vi "Target4.vi"   [LabVIEW 2025]
uses:
  <vilib>/eio/utilities/niEioResolveVilibRelativePath.vi
  <vilib>/rvi/interface/RandomDataEmulation/niFpgaRandomDataHandleErrors.vi
  <vilib>/rvi/Memory/Memory_Emulation/nirvimemoryFastEmulation.vi
  <vilib>/rvi/Memory/Memory_Emulation/nirvimemoryEmulation.vi
  <vilib>/rvi/Emulation/niFpgaEmulationIsFPGAContextNoSignature.vi
  <vilib>/rvi/DataTransferAndStorage/Container/Common/niFpgaContainerGetUniqueNameForEmu.vi
  <vilib>/rvi/Emulation/niFpgaProcessEmulError.vi
  <vilib>/rvi/Emulation/niFpgaSctlEmulationGetInTimedLoop.vi
  <vilib>/rvi/errors/nirviReportUnexpectedCaseInternalError (U32).vi
  <vilib>/rvi/DataTransferAndStorage/Container/XNode/niFpgaContainer.xnode
  <vilib>/rvi/interface/RandomDataEmulation/nirviRandomDataFpgaReadWriteTemplate.vi
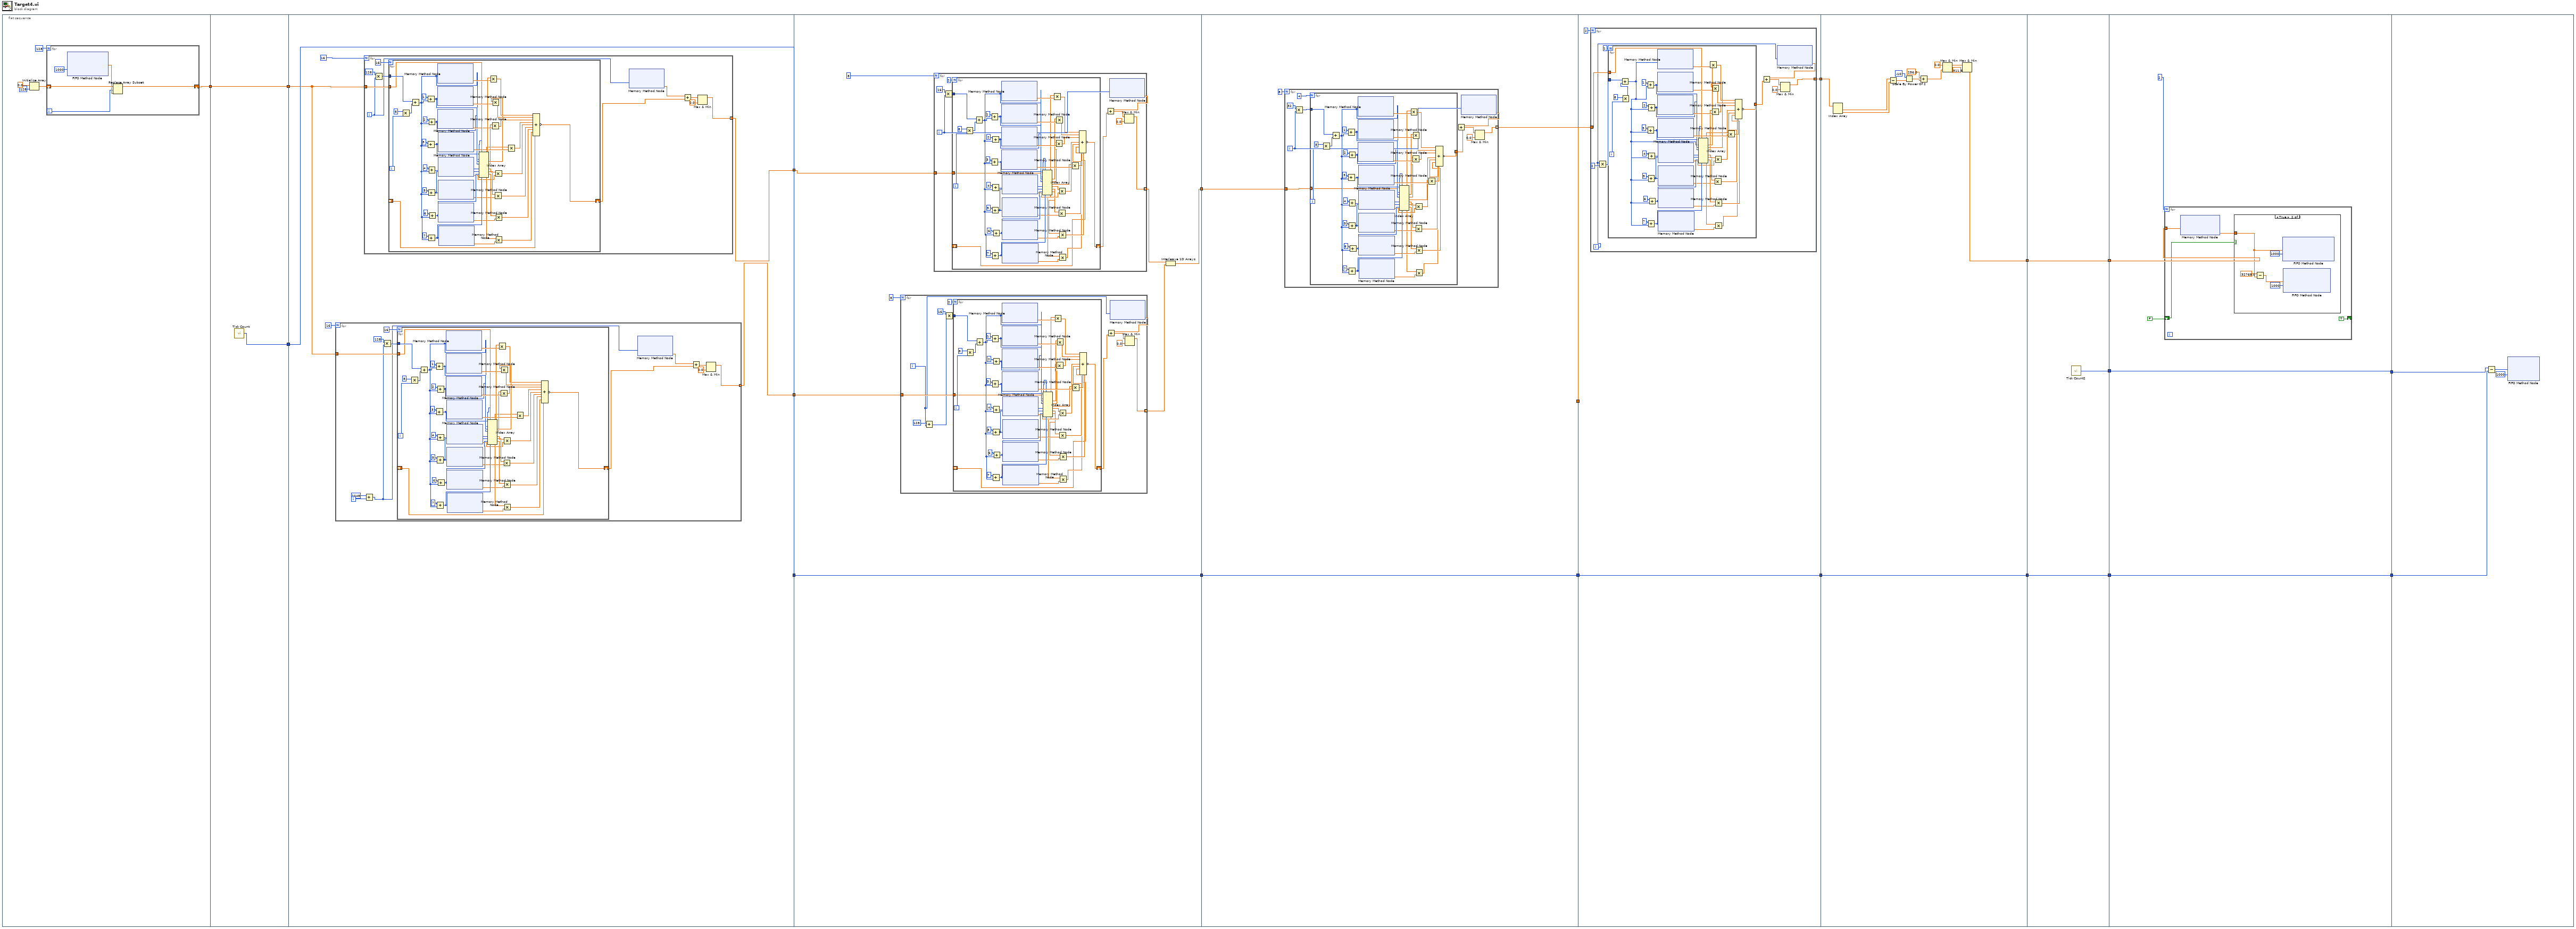
[diagram p0: block diagram]
diagram:
  n1 = flat-sequence {
    tunnel: [w23] -> w19
    tunnel: w19 -> [w31]
    tunnel: [w31] -> w18
    tunnel: [w30] -> w17
    tunnel: w18 -> [w34]
    tunnel: w17 -> [w36]
    tunnel: [w36] -> w7
    tunnel: [w33] -> w2
    tunnel: [w32] -> w1
    tunnel: w7 -> [w159]
    tunnel: [w159] -> w5
    tunnel: [w156] -> w3
    tunnel: w2 -> [w153]
    tunnel: w1 -> [w152]
    tunnel: [w275] -> w6
    tunnel: w5 -> [w277]
    tunnel: [w277] -> w4
    tunnel: w3 -> [w274]
    tunnel: w6 -> [w335]
    tunnel: [w334] -> w16
    tunnel: [w336] -> w8
    tunnel: w4 -> [w336]
    tunnel: w16 -> [w394]
    tunnel: [w396] -> w15
    tunnel: [w395] -> w9
    tunnel: w8 -> [w395]
    tunnel: w15 -> [w407]
    tunnel: [w407] -> w14
    tunnel: [w406] -> w13
    tunnel: [w405] -> w10
    tunnel: w9 -> [w405]
    tunnel: w14 -> [w411]
    tunnel: [w409] -> w12
    tunnel: w13 -> [w409]
    tunnel: [w408] -> w11
    tunnel: w10 -> [w408]
    tunnel: w12 -> [w425]
    tunnel: w11 -> [w422]
    frame #0 {
      n2 = Initialize Array(sgl 0.0 ("element"), 128 ("dimension size")) -> (w20:sgl[])
      n3 = for {
        N: 128 -> [_]
        shift-right: [w26] -> w23
        shift-left: w20 -> [w28]
        i -> [w25]
        n4 = xnode ("FIFO Method Node")("Timeout"=1000) -> ("Element"=w27:sgl)  [unwired: 1 in, 2 out]
        n5 = Replace Array Subset(array=w28, new element=w27, index=w25) -> (w26:sgl[])
      }
    }
    frame #1 {
      n6 = call "Tick Count"() -> ("Tick Count(uSec)"=w30:u32)
    }
    frame #2 {
      n7 = for {
        N: 16 -> [_]
        tunnel: w34 -> [w44]
        tunnel: [w43] -> w32 mode=indexing
        i -> [w40]
        n8 = Add(x=2048, y=w40) -> (x+y=w39:i32)
        n9 = Multiply(x=128, y=w39) -> (x*y=w47:i32)
        n10 = for {
          N: 16 -> [_]
          tunnel: w47 -> [w95]
          tunnel: w44 -> [w81]
          shift-right: [w50] -> w42
          shift-left: _ -> [w51]
          i -> [w94]
          n11 = Multiply(x=8, y=w94) -> (x*y=w92:i32)
          n12 = Add(x=w95, y=w92) -> (x+y=w56:i32)
          n13 = Add(x=1, y=w56) -> (x+y=w78:i32)
          n14 = Add(x=3, y=w56) -> (x+y=w74:i32)
          n15 = Add(x=5, y=w56) -> (x+y=w67:i32)
          n16 = Add(x=7, y=w56) -> (x+y=w65:i32)
          n17 = Add(x=2, y=w56) -> (x+y=w73:i32)
          n18 = Add(x=4, y=w56) -> (x+y=w68:i32)
          n19 = Add(x=6, y=w56) -> (x+y=w66:i32)
          n20 = xnode ("Memory Method Node")("Address"=w56) -> ("Data"=w87:sgl)  [unwired: 1 in, 1 out]
          n21 = xnode ("Memory Method Node")("Address"=w78) -> ("Data"=w82:sgl)  [unwired: 1 in, 1 out]
          n22 = xnode ("Memory Method Node")("Address"=w73) -> ("Data"=w79:sgl)  [unwired: 1 in, 1 out]
          n23 = xnode ("Memory Method Node")("Address"=w74) -> ("Data"=w80:sgl)  [unwired: 1 in, 1 out]
          n24 = xnode ("Memory Method Node")("Address"=w68) -> ("Data"=w57:sgl)  [unwired: 1 in, 1 out]
          n25 = xnode ("Memory Method Node")("Address"=w67) -> ("Data"=w58:sgl)  [unwired: 1 in, 1 out]
          n26 = xnode ("Memory Method Node")("Address"=w66) -> ("Data"=w59:sgl)  [unwired: 1 in, 1 out]
          n27 = xnode ("Memory Method Node")("Address"=w65) -> ("Data"=w60:sgl)  [unwired: 1 in, 1 out]
          n28 = Index Array(array=w81, index #1=w56, index #2=w78, index #3=w73, index #4=w74, index #5=w68, index #6=w67, index #7=w66, index #8=w65) -> (element #1=w88:sgl, element #2=w77:sgl, element #3=w76:sgl, element #4=w75:sgl, element #5=w64:sgl, element #6=w63:sgl, element #7=w62:sgl, element #8=w61:sgl)
          n29 = Multiply(x=w88, y=w87) -> (x*y=w86:sgl)
          n30 = Multiply(x=w76, y=w79) -> (x*y=w84:sgl)
          n31 = Multiply(x=w77, y=w82) -> (x*y=w85:sgl)
          n32 = Multiply(x=w63, y=w58) -> (x*y=w54:sgl)
          n33 = Multiply(x=w64, y=w57) -> (x*y=w55:sgl)
          n34 = Multiply(x=w62, y=w59) -> (x*y=w53:sgl)
          n35 = Multiply(x=w61, y=w60) -> (x*y=w52:sgl)
          n36 = Multiply(x=w75, y=w80) -> (x*y=w83:sgl)
          n37 = Compound Arithmetic op=ADD(w86, w85, w84, w83, w55, w54, w53, w52, w51) -> (invert w50:sgl)
        }
        n38 = xnode ("Memory Method Node")("Address"=w39) -> ("Data"=w41:sgl)  [unwired: 1 in, 1 out]
        n39 = Add(x=w41, y=w42) -> (x+y=w46:sgl)
        n40 = Max & Min(x=w46, y=sgl 0.0) -> (max(x,y)=w43:sgl)  [unwired: 1 out]
      }
      n41 = for {
        N: 16 -> [_]
        tunnel: w34 -> [w100]
        tunnel: [w98] -> w33 mode=indexing
        i -> [w99]
        n42 = Multiply(x=128, y=w99) -> (x*y=w103:i32)
        n43 = for {
          N: 16 -> [_]
          tunnel: w103 -> [w151]
          tunnel: w100 -> [w137]
          shift-right: [w106] -> w97
          shift-left: _ -> [w107]
          i -> [w150]
          n44 = Multiply(x=8, y=w150) -> (x*y=w148:i32)
          n45 = Add(x=w151, y=w148) -> (x+y=w112:i32)
          n46 = Add(x=1, y=w112) -> (x+y=w134:i32)
          n47 = Add(x=3, y=w112) -> (x+y=w130:i32)
          n48 = Add(x=5, y=w112) -> (x+y=w123:i32)
          n49 = Add(x=7, y=w112) -> (x+y=w121:i32)
          n50 = Add(x=2, y=w112) -> (x+y=w129:i32)
          n51 = Add(x=4, y=w112) -> (x+y=w124:i32)
          n52 = Add(x=6, y=w112) -> (x+y=w122:i32)
          n53 = xnode ("Memory Method Node")("Address"=w112) -> ("Data"=w143:sgl)  [unwired: 1 in, 1 out]
          n54 = xnode ("Memory Method Node")("Address"=w134) -> ("Data"=w138:sgl)  [unwired: 1 in, 1 out]
          n55 = xnode ("Memory Method Node")("Address"=w129) -> ("Data"=w135:sgl)  [unwired: 1 in, 1 out]
          n56 = xnode ("Memory Method Node")("Address"=w130) -> ("Data"=w136:sgl)  [unwired: 1 in, 1 out]
          n57 = xnode ("Memory Method Node")("Address"=w124) -> ("Data"=w113:sgl)  [unwired: 1 in, 1 out]
          n58 = xnode ("Memory Method Node")("Address"=w123) -> ("Data"=w114:sgl)  [unwired: 1 in, 1 out]
          n59 = xnode ("Memory Method Node")("Address"=w122) -> ("Data"=w115:sgl)  [unwired: 1 in, 1 out]
          n60 = xnode ("Memory Method Node")("Address"=w121) -> ("Data"=w116:sgl)  [unwired: 1 in, 1 out]
          n61 = Index Array(array=w137, index #1=w112, index #2=w134, index #3=w129, index #4=w130, index #5=w124, index #6=w123, index #7=w122, index #8=w121) -> (element #1=w144:sgl, element #2=w133:sgl, element #3=w132:sgl, element #4=w131:sgl, element #5=w120:sgl, element #6=w119:sgl, element #7=w118:sgl, element #8=w117:sgl)
          n62 = Multiply(x=w144, y=w143) -> (x*y=w142:sgl)
          n63 = Multiply(x=w132, y=w135) -> (x*y=w140:sgl)
          n64 = Multiply(x=w133, y=w138) -> (x*y=w141:sgl)
          n65 = Multiply(x=w119, y=w114) -> (x*y=w110:sgl)
          n66 = Multiply(x=w120, y=w113) -> (x*y=w111:sgl)
          n67 = Multiply(x=w118, y=w115) -> (x*y=w109:sgl)
          n68 = Multiply(x=w117, y=w116) -> (x*y=w108:sgl)
          n69 = Multiply(x=w131, y=w136) -> (x*y=w139:sgl)
          n70 = Compound Arithmetic op=ADD(w142, w141, w140, w139, w111, w110, w109, w108, w107) -> (invert w106:sgl)
        }
        n71 = xnode ("Memory Method Node")("Address"=w99) -> ("Data"=w96:sgl)  [unwired: 1 in, 1 out]
        n72 = Add(x=w96, y=w97) -> (x+y=w102:sgl)
        n73 = Max & Min(x=w102, y=sgl 0.0) -> (max(x,y)=w98:sgl)  [unwired: 1 out]
      }
    }
    frame #3 {
      n74 = for {
        N: 8 -> [_]
        tunnel: w152 -> [w165]
        tunnel: [w164] -> w154 mode=indexing
        i -> [w160]
        n75 = Add(x=128, y=w160) -> (x+y=w161:i32)
        n76 = Multiply(x=16, y=w161) -> (x*y=w168:i32)
        n77 = for {
          N: 2 -> [_]
          tunnel: w168 -> [w217]
          tunnel: w165 -> [w182]
          shift-right: [w173] -> w163
          shift-left: _ -> [w172]
          i -> [w216]
          n78 = Multiply(x=8, y=w216) -> (x*y=w214:i32)
          n79 = Add(x=w217, y=w214) -> (x+y=w183:i32)
          n80 = Add(x=1, y=w183) -> (x+y=w202:i32)
          n81 = Add(x=3, y=w183) -> (x+y=w201:i32)
          n82 = Add(x=5, y=w183) -> (x+y=w194:i32)
          n83 = Add(x=7, y=w183) -> (x+y=w192:i32)
          n84 = Add(x=2, y=w183) -> (x+y=w200:i32)
          n85 = Add(x=4, y=w183) -> (x+y=w195:i32)
          n86 = Add(x=6, y=w183) -> (x+y=w193:i32)
          n87 = xnode ("Memory Method Node")("Address"=w183) -> ("Data"=w210:sgl)  [unwired: 1 in, 1 out]
          n88 = xnode ("Memory Method Node")("Address"=w202) -> ("Data"=w205:sgl)  [unwired: 1 in, 1 out]
          n89 = xnode ("Memory Method Node")("Address"=w200) -> ("Data"=w203:sgl)  [unwired: 1 in, 1 out]
          n90 = xnode ("Memory Method Node")("Address"=w201) -> ("Data"=w204:sgl)  [unwired: 1 in, 1 out]
          n91 = xnode ("Memory Method Node")("Address"=w195) -> ("Data"=w188:sgl)  [unwired: 1 in, 1 out]
          n92 = xnode ("Memory Method Node")("Address"=w194) -> ("Data"=w189:sgl)  [unwired: 1 in, 1 out]
          n93 = xnode ("Memory Method Node")("Address"=w193) -> ("Data"=w190:sgl)  [unwired: 1 in, 1 out]
          n94 = xnode ("Memory Method Node")("Address"=w192) -> ("Data"=w191:sgl)  [unwired: 1 in, 1 out]
          n95 = Index Array(array=w182, index #1=w183, index #2=w202, index #3=w200, index #4=w201, index #5=w195, index #6=w194, index #7=w193, index #8=w192) -> (element #1=w181:sgl, element #2=w180:sgl, element #3=w179:sgl, element #4=w177:sgl, element #5=w178:sgl, element #6=w176:sgl, element #7=w175:sgl, element #8=w174:sgl)
          n96 = Multiply(x=w181, y=w210) -> (x*y=w209:sgl)
          n97 = Multiply(x=w179, y=w203) -> (x*y=w207:sgl)
          n98 = Multiply(x=w180, y=w205) -> (x*y=w208:sgl)
          n99 = Multiply(x=w176, y=w189) -> (x*y=w186:sgl)
          n100 = Multiply(x=w178, y=w188) -> (x*y=w187:sgl)
          n101 = Multiply(x=w175, y=w190) -> (x*y=w185:sgl)
          n102 = Multiply(x=w174, y=w191) -> (x*y=w184:sgl)
          n103 = Multiply(x=w177, y=w204) -> (x*y=w206:sgl)
          n104 = Compound Arithmetic op=ADD(w209, w208, w207, w206, w187, w186, w185, w184, w172) -> (invert w173:sgl)
        }
        n105 = xnode ("Memory Method Node")("Address"=w160) -> ("Data"=w170:sgl)  [unwired: 1 in, 1 out]
        n106 = Add(x=w170, y=w163) -> (x+y=w167:sgl)
        n107 = Max & Min(x=w167, y=sgl 0.0) -> (max(x,y)=w164:sgl)  [unwired: 1 out]
      }
      n108 = for {
        N: 8 -> [_]
        tunnel: w153 -> [w220]
        tunnel: [w219] -> w155 mode=indexing
        i -> [w224]
        n109 = Multiply(x=16, y=w224) -> (x*y=w223:i32)
        n110 = for {
          N: 2 -> [_]
          tunnel: w223 -> [w273]
          tunnel: w220 -> [w238]
          shift-right: [w229] -> w218
          shift-left: _ -> [w228]
          i -> [w272]
          n111 = Multiply(x=8, y=w272) -> (x*y=w270:i32)
          n112 = Add(x=w273, y=w270) -> (x+y=w239:i32)
          n113 = Add(x=1, y=w239) -> (x+y=w258:i32)
          n114 = Add(x=3, y=w239) -> (x+y=w257:i32)
          n115 = Add(x=5, y=w239) -> (x+y=w250:i32)
          n116 = Add(x=7, y=w239) -> (x+y=w248:i32)
          n117 = Add(x=2, y=w239) -> (x+y=w256:i32)
          n118 = Add(x=4, y=w239) -> (x+y=w251:i32)
          n119 = Add(x=6, y=w239) -> (x+y=w249:i32)
          n120 = xnode ("Memory Method Node")("Address"=w239) -> ("Data"=w266:sgl)  [unwired: 1 in, 1 out]
          n121 = xnode ("Memory Method Node")("Address"=w258) -> ("Data"=w261:sgl)  [unwired: 1 in, 1 out]
          n122 = xnode ("Memory Method Node")("Address"=w256) -> ("Data"=w259:sgl)  [unwired: 1 in, 1 out]
          n123 = xnode ("Memory Method Node")("Address"=w257) -> ("Data"=w260:sgl)  [unwired: 1 in, 1 out]
          n124 = xnode ("Memory Method Node")("Address"=w251) -> ("Data"=w244:sgl)  [unwired: 1 in, 1 out]
          n125 = xnode ("Memory Method Node")("Address"=w250) -> ("Data"=w245:sgl)  [unwired: 1 in, 1 out]
          n126 = xnode ("Memory Method Node")("Address"=w249) -> ("Data"=w246:sgl)  [unwired: 1 in, 1 out]
          n127 = xnode ("Memory Method Node")("Address"=w248) -> ("Data"=w247:sgl)  [unwired: 1 in, 1 out]
          n128 = Index Array(array=w238, index #1=w239, index #2=w258, index #3=w256, index #4=w257, index #5=w251, index #6=w250, index #7=w249, index #8=w248) -> (element #1=w237:sgl, element #2=w236:sgl, element #3=w235:sgl, element #4=w233:sgl, element #5=w234:sgl, element #6=w232:sgl, element #7=w231:sgl, element #8=w230:sgl)
          n129 = Multiply(x=w237, y=w266) -> (x*y=w265:sgl)
          n130 = Multiply(x=w235, y=w259) -> (x*y=w263:sgl)
          n131 = Multiply(x=w236, y=w261) -> (x*y=w264:sgl)
          n132 = Multiply(x=w232, y=w245) -> (x*y=w242:sgl)
          n133 = Multiply(x=w234, y=w244) -> (x*y=w243:sgl)
          n134 = Multiply(x=w231, y=w246) -> (x*y=w241:sgl)
          n135 = Multiply(x=w230, y=w247) -> (x*y=w240:sgl)
          n136 = Multiply(x=w233, y=w260) -> (x*y=w262:sgl)
          n137 = Compound Arithmetic op=ADD(w265, w264, w263, w262, w243, w242, w241, w240, w228) -> (invert w229:sgl)
        }
        n138 = xnode ("Memory Method Node")("Address"=w224) -> ("Data"=w226:sgl)  [unwired: 1 in, 1 out]
        n139 = Add(x=w226, y=w218) -> (x+y=w222:sgl)
        n140 = Max & Min(x=w222, y=sgl 0.0) -> (max(x,y)=w219:sgl)  [unwired: 1 out]
      }
      n141 = Interleave 1D Arrays(w155, w154) -> (w156:sgl[])
    }
    frame #4 {
      n142 = for {
        N: 8 -> [_]
        tunnel: [w280] -> w275 mode=indexing
        tunnel: w274 -> [w278]
        i -> [w284]
        n143 = Multiply(x=32, y=w284) -> (x*y=w283:i32)
        n144 = for {
          N: 4 -> [_]
          tunnel: w283 -> [w332]
          tunnel: [w317] -> w279
          tunnel: w278 -> [w296]
          i -> [w331]
          n145 = Multiply(x=8, y=w331) -> (x*y=w329:i32)
          n146 = Add(x=w332, y=w329) -> (x+y=w297:i32)
          n147 = Add(x=1, y=w297) -> (x+y=w316:i32)
          n148 = Add(x=3, y=w297) -> (x+y=w315:i32)
          n149 = Add(x=5, y=w297) -> (x+y=w308:i32)
          n150 = Add(x=7, y=w297) -> (x+y=w306:i32)
          n151 = Add(x=2, y=w297) -> (x+y=w314:i32)
          n152 = Add(x=4, y=w297) -> (x+y=w309:i32)
          n153 = Add(x=6, y=w297) -> (x+y=w307:i32)
          n154 = xnode ("Memory Method Node")("Address"=w297) -> ("Data"=w325:sgl)  [unwired: 1 in, 1 out]
          n155 = xnode ("Memory Method Node")("Address"=w316) -> ("Data"=w320:sgl)  [unwired: 1 in, 1 out]
          n156 = xnode ("Memory Method Node")("Address"=w314) -> ("Data"=w318:sgl)  [unwired: 1 in, 1 out]
          n157 = xnode ("Memory Method Node")("Address"=w315) -> ("Data"=w319:sgl)  [unwired: 1 in, 1 out]
          n158 = xnode ("Memory Method Node")("Address"=w309) -> ("Data"=w302:sgl)  [unwired: 1 in, 1 out]
          n159 = xnode ("Memory Method Node")("Address"=w308) -> ("Data"=w303:sgl)  [unwired: 1 in, 1 out]
          n160 = xnode ("Memory Method Node")("Address"=w307) -> ("Data"=w304:sgl)  [unwired: 1 in, 1 out]
          n161 = xnode ("Memory Method Node")("Address"=w306) -> ("Data"=w305:sgl)  [unwired: 1 in, 1 out]
          n162 = Index Array(array=w296, index #1=w297, index #2=w316, index #3=w314, index #4=w315, index #5=w309, index #6=w308, index #7=w307, index #8=w306) -> (element #1=w295:sgl, element #2=w294:sgl, element #3=w293:sgl, element #4=w292:sgl, element #5=w291:sgl, element #6=w290:sgl, element #7=w289:sgl, element #8=w288:sgl)
          n163 = Multiply(x=w295, y=w325) -> (x*y=w324:sgl)
          n164 = Multiply(x=w293, y=w318) -> (x*y=w322:sgl)
          n165 = Multiply(x=w294, y=w320) -> (x*y=w323:sgl)
          n166 = Multiply(x=w290, y=w303) -> (x*y=w300:sgl)
          n167 = Multiply(x=w291, y=w302) -> (x*y=w301:sgl)
          n168 = Multiply(x=w289, y=w304) -> (x*y=w299:sgl)
          n169 = Multiply(x=w288, y=w305) -> (x*y=w298:sgl)
          n170 = Multiply(x=w292, y=w319) -> (x*y=w321:sgl)
          n171 = Compound Arithmetic op=ADD(w324, w323, w322, w321, w301, w300, w299, w298) -> (invert w317:sgl)
        }
        n172 = xnode ("Memory Method Node")("Address"=w284) -> ("Data"=w286:sgl)  [unwired: 1 in, 1 out]
        n173 = Add(x=w286, y=w279) -> (x+y=w282:sgl)
        n174 = Max & Min(x=w282, y=sgl 0.0) -> (max(x,y)=w280:sgl)  [unwired: 1 out]
      }
    }
    frame #5 {
      n175 = for {
        N: 2 -> [_]
        tunnel: w335 -> [w346]
        tunnel: [w345] -> w334 mode=indexing
        i -> [w337]
        n176 = Multiply(x=w337, y=2) -> (x*y=w338:i32)
        n177 = for {
          N: 1 -> [_]
          tunnel: w346 -> [w379]
          tunnel: [w376] -> w340
          tunnel: w338 -> [w347]
          i -> [w391]
          n178 = Multiply(x=8, y=w391) -> (x*y=w349:i32)
          n179 = Add(x=w347, y=w349) -> (x+y=w348:i32)
          n180 = Add(x=1, y=w348) -> (x+y=w375:i32)
          n181 = Add(x=3, y=w348) -> (x+y=w371:i32)
          n182 = Add(x=5, y=w348) -> (x+y=w364:i32)
          n183 = Add(x=7, y=w348) -> (x+y=w362:i32)
          n184 = Add(x=2, y=w348) -> (x+y=w370:i32)
          n185 = Add(x=4, y=w348) -> (x+y=w365:i32)
          n186 = Add(x=6, y=w348) -> (x+y=w363:i32)
          n187 = xnode ("Memory Method Node")("Address"=w348) -> ("Data"=w385:sgl)  [unwired: 1 in, 1 out]
          n188 = xnode ("Memory Method Node")("Address"=w375) -> ("Data"=w380:sgl)  [unwired: 1 in, 1 out]
          n189 = xnode ("Memory Method Node")("Address"=w370) -> ("Data"=w377:sgl)  [unwired: 1 in, 1 out]
          n190 = xnode ("Memory Method Node")("Address"=w371) -> ("Data"=w378:sgl)  [unwired: 1 in, 1 out]
          n191 = xnode ("Memory Method Node")("Address"=w365) -> ("Data"=w354:sgl)  [unwired: 1 in, 1 out]
          n192 = xnode ("Memory Method Node")("Address"=w364) -> ("Data"=w355:sgl)  [unwired: 1 in, 1 out]
          n193 = xnode ("Memory Method Node")("Address"=w363) -> ("Data"=w356:sgl)  [unwired: 1 in, 1 out]
          n194 = xnode ("Memory Method Node")("Address"=w362) -> ("Data"=w357:sgl)  [unwired: 1 in, 1 out]
          n195 = Index Array(array=w379, index #1=w348, index #2=w375, index #3=w370, index #4=w371, index #5=w365, index #6=w364, index #7=w363, index #8=w362) -> (element #1=w386:sgl, element #2=w374:sgl, element #3=w373:sgl, element #4=w372:sgl, element #5=w361:sgl, element #6=w360:sgl, element #7=w359:sgl, element #8=w358:sgl)
          n196 = Multiply(x=w386, y=w385) -> (x*y=w384:sgl)
          n197 = Multiply(x=w373, y=w377) -> (x*y=w382:sgl)
          n198 = Multiply(x=w374, y=w380) -> (x*y=w383:sgl)
          n199 = Multiply(x=w360, y=w355) -> (x*y=w352:sgl)
          n200 = Multiply(x=w361, y=w354) -> (x*y=w353:sgl)
          n201 = Multiply(x=w359, y=w356) -> (x*y=w351:sgl)
          n202 = Multiply(x=w358, y=w357) -> (x*y=w350:sgl)
          n203 = Multiply(x=w372, y=w378) -> (x*y=w381:sgl)
          n204 = Compound Arithmetic op=ADD(w384, w383, w382, w381, w353, w352, w351, w350) -> (invert w376:sgl)
        }
        n205 = xnode ("Memory Method Node")("Address"=w337) -> ("Data"=w343:sgl)  [unwired: 1 in, 1 out]
        n206 = Add(x=w343, y=w340) -> (x+y=w342:sgl)
        n207 = Max & Min(x=w342, y=sgl 0.0) -> (max(x,y)=w345:sgl)  [unwired: 1 out]
      }
    }
    frame #6 {
      n208 = Index Array(array=w394) -> (element #1=w393:sgl, element #2=w392:sgl)  [unwired: 2 in]
      n209 = Subtract(x=w393, y=w392) -> (x-y=w401:sgl)
      n210 = Scale By Power Of 2(n=i16 -10, x=w401) -> (x*2^n=w402:sgl)
      n211 = Add(x=sgl 256.0, y=w402) -> (x+y=w403:sgl)
      n212 = Max & Min(x=sgl 0.0, y=w403) -> (max(x,y)=w404:sgl)  [unwired: 1 out]
      n213 = Max & Min(x=w404, y=sgl 511.0) -> (min(x,y)=w396:sgl)  [unwired: 1 out]
    }
    frame #7 {
      n214 = call "Tick Count2"() -> ("Tick Count(uSec)"=w406:u32)
    }
    frame #8 {
      n215 = for {
        N: 2 -> [_]
        tunnel: w411 -> [w416]
        shift-right: [TRUE] -> _
        shift-left: FALSE -> [w415]
        n216 = xnode ("Memory Method Node")("Address"=w416) -> ("Data"=w413:sgl)  [unwired: 1 in, 1 out]
        n217 = case shown="True" w415 {
          tunnel: w413 -> [_ w417]
          frame False {
          }
          frame True {
            n218 = Subtract(x=sgl 32768.0, y=w417) -> (x-y=w421:sgl)
            n219 = xnode ("FIFO Method Node")("Element"=w417, "Timeout"=1000) -> ()  [unwired: 1 in, 2 out]
            n220 = xnode ("FIFO Method Node")("Element"=w421, "Timeout"=1000) -> ()  [unwired: 1 in, 2 out]
          }
        }
      }
    }
    frame #9 {
      n221 = Subtract(x=w425, y=w422) -> (x-y=w424:u32)
      n222 = xnode ("FIFO Method Node")("Element"=w424, "Timeout"=1000) -> ()  [unwired: 1 in, 2 out]
    }
  }
